vi "PID.vi"(6 "Reinit":bool, 7 "Gains":T1, 8 "dT":dbl, 10 "Current":dbl, 11 "Target":dbl) -> (3 "Out":dbl)   [LabVIEW 2020]
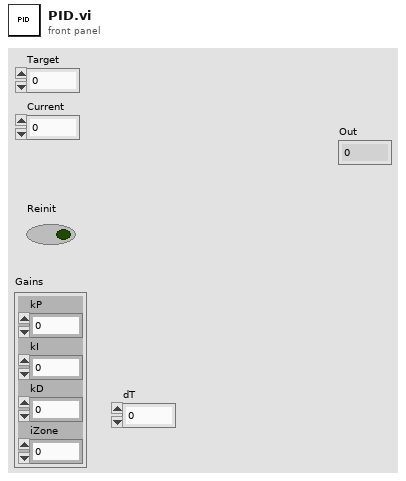
[diagram p1: front panel]
types:
  T1 = cluster{"kP":dbl, "kI":dbl, "kD":dbl, "iZone":dbl}
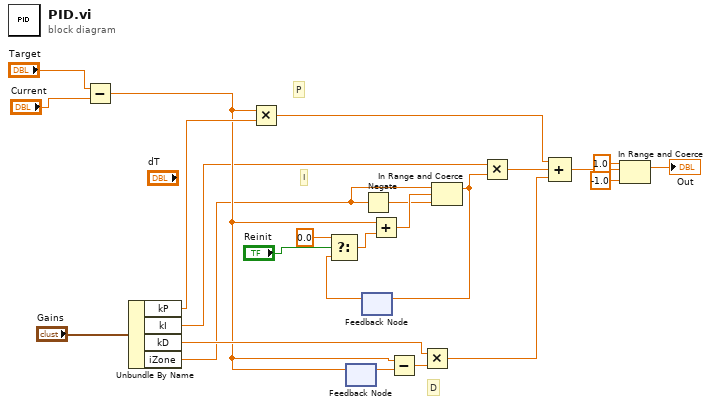
[diagram p0: block diagram]
diagram:
  # "D"
  # "I"
  # "P"
  n1 = Subtract(x="Target", y="Current") -> (x-y=w6:dbl)
  n2 = Unbundle By Name("Gains") -> ("kP"=w18:dbl, "kI"=w5:dbl, "kD"=w11:dbl, "iZone"=w2:dbl)
  n3 = Multiply(x=w6, y=w18) -> (x*y=w9:dbl)
  n4 = feedback-in #1(w6) -> ()
  n5 = feedback #1() -> (w13:dbl)  [unwired: 1 in]
  n6 = feedback #2() -> (w16:dbl)  [unwired: 1 in]
  n7 = Select(t=0.0, s="Reinit", f=w16) -> (s? t:f=w15:dbl)
  n8 = Negate(x=w2) -> (-x=w3:dbl)
  n9 = Add(x=w6, y=w15) -> (x+y=w4:dbl)
  n10 = Subtract(x=w6, y=w13) -> (x-y=w12:dbl)
  n11 = Multiply(x=w11, y=w12) -> (x*y=w8:dbl)
  n12 = In Range and Coerce(upper limit=w2, x=w4, lower limit=w3) -> (coerced(x)=w1:dbl)  [unwired: 1 out]
  n13 = feedback-in #2(w1) -> ()
  n14 = Multiply(x=w5, y=w1) -> (x*y=w7:dbl)
  n15 = Compound Arithmetic op=ADD(w9, w7, w8) -> (w10:dbl)
  n16 = In Range and Coerce(upper limit=1.0, x=w10, lower limit=-1.0) -> (coerced(x)=→"Out":dbl)  [unwired: 1 out]
